vi "Read State.vi"(8 "error in (no error)":errorcluster, 11 "Switch in":refnum<class "Switch.lvclass">) -> (0 "error out":errorcluster, 2 "State":bool, 3 "Switch out":refnum<class "Switch.lvclass">)   [LabVIEW 2015, in "Switch.lvclass"]
uses:
  Switch.lvclass
  Switch.lvclass/Switch.ctl
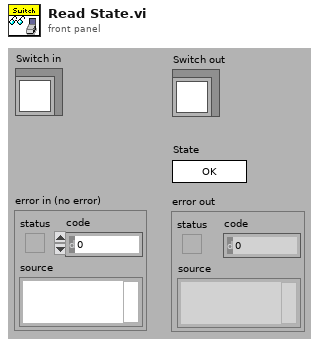
[diagram p1: front panel]
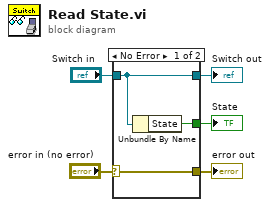
[diagram p0: block diagram]
diagram:
  n1 = case shown="No Error" "error in (no error)" {
    selector: "error in (no error)" -> [w8 w9]
    tunnel: [w8 w9] -> w4
    tunnel: [w7 w10] -> w2
    tunnel: "Switch in" -> [w7 w10]
    tunnel: [w6 _] -> w1
    frame No Error {
      n2 = Unbundle By Name(w7) -> ("State"=w6:bool)
    }
    frame Error {
    }
  }
  "error out" <- w4
  "Switch out" <- w2
  "State" <- w1
